vi "dfd_Cosine Modulated Coefficients Combine States and Input.vi"(8 "number of bands":i32, 9 "coeff":dbl[](array[numeric]), 10 "states in":dbl[][](array[numeric]), 11 "x":dbl[][](array[numeric])) -> (0 "2m-1":i32, 3 "y":dbl[][](array[numeric]))   [LabVIEW 2017, in "NI_DigFilter_FilterBank.lvlib"]
uses:
  <vilib>/addons/Digital Filter Design/NI_DigFilter_FilterBank.lvlib
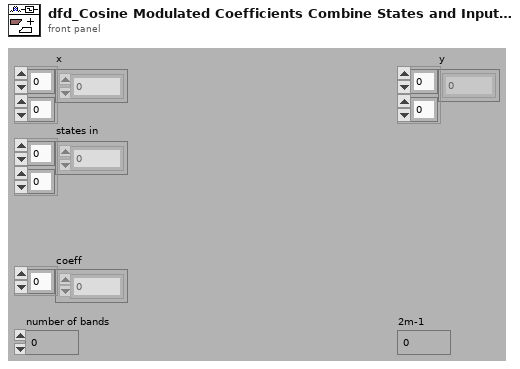
[diagram p1: front panel]
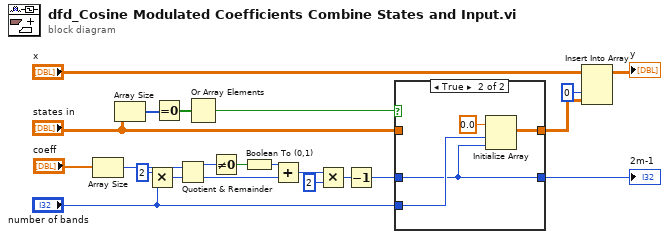
[diagram p0: block diagram]
diagram:
  n1 = Array Size(array="coeff") -> (size(s)=w9:i32)
  n2 = Array Size(array="states in") -> (size(s)=w18:i32[])
  n3 = Multiply(x=2 ("y"), y="number of bands") -> (x*y=w17:i32)
  n4 = Equal To 0?(x=w18) -> (x = 0?=w21:bool[])
  n5 = Quotient & Remainder(x=w9, y=w17) -> (x-y*floor(x/y)=w16:i32, floor(x/y)=w13:i32)
  n6 = Or Array Elements(Boolean array=w21) -> (logical OR=w22:bool)
  n7 = Not Equal To 0?(x=w16) -> (x != 0?=w15:bool)
  n8 = Boolean To (0,1)(Boolean=w15) -> (0, 1=w14:i16)
  n9 = Add(x=w14, y=w13) -> (x+y=w11:i32)
  n10 = Multiply(x=w11, y=2) -> (x*y=w10:i32)
  n11 = Decrement(x=w10) -> (x-1=w5:i32)
  n12 = case shown="True" w22 {
    tunnel: "states in" -> [w24 _]
    tunnel: [w24 w28] -> w20
    tunnel: "number of bands" -> [_ w26]
    tunnel: w5 -> [w23 w25]
    tunnel: [w23 w25] -> w4
    frame False {
    }
    frame True {
      n13 = Initialize Array(0.0 ("element"), w26, w25) -> (w28:dbl[][])
    }
  }
  "2m-1" <- w4
  n14 = Insert Into Array(array="x", index (col)=0 ("disabled index (col)"), new element=w20) -> (→"y":dbl[][])  [unwired: 1 in]
